vi "DMM6500_Soft_v0.vi"() -> ()   [LabVIEW 2023]
uses:
  Ctrl_state.ctl
  <vilib>/Instr/_visa.llb/VISA Find Search Mode.ctl
  <vilib>/Instr/_visa.llb/VISA Open Access Mode.ctl
  <vilib>/Utility/sysdir.llb/System Directory Type.ctl
  <instrlib>/Keithley DMM6500 DAQ6500 Series/Public/Data/Read (Multiple Points).vi
  <instrlib>/Keithley DMM6500 DAQ6500 Series/Keithley DMM6500 DAQ6500 Series.lvlib
panel:
  in  "Manual Range (1)":dbl=1.0 format="%#_13g"
  in  "Auto Range":bool=TRUE
  in  "Label":string="Sensor label"
  in  "NPLC":dbl(ring)=10.0 items=["0.01"=0.01, "0.1"=0.1, "1"=1.0, "5"=5.0, "10"=10.0, "25"=25.0, "50"=50.0]
  in  "Function (0: Voltage DC)":i32(ring)=4 items=["Voltage DC", "Voltage AC", "Current DC", "Current AC", "Resistance", "4-wire Resistance", "Diode", "Capacitance", "Temperature", "Continuity", "Frequency", "Period", "Voltage Ratio", "Digitize Voltage", "Digitize Current"]
  in  "Sensors":T1(array[cluster])
  in  "Meas":bool
  in  "Stop":bool
  out "Status":string
  out "Err/MSG":string
  in  "Tab Control":enum32{"Time Domain"}(tab)
  out "Data":cluster{dbl[], dbl[]}[](graph)
  # "Martin Hruska, 2026"
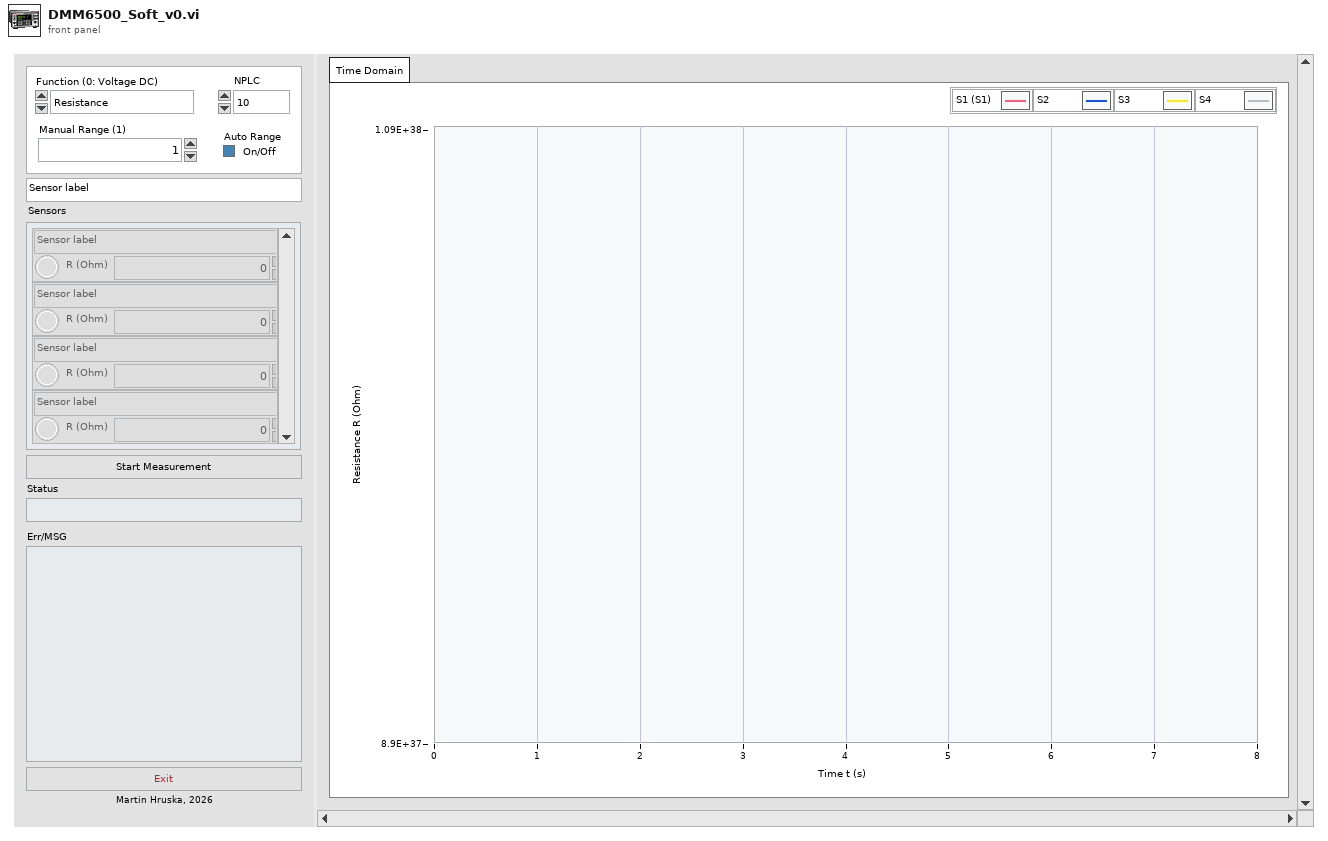
[diagram p1: front panel]
types:
  T1 = cluster{"S Label":string, "S On/Off":bool, "R (Ohm)":dbl}[]
  T2 = typedef "Ctrl_state.ctl" = enum16{"Initialize", "Wait", "Close", "Continuous"}
  T3 = enum8{"Enabled", "Disabled", "Disabled and Grayed Out"}
  T4 = enum16{"open", "replace", "create", "open or create", "replace or create", "replace or create with confirmation"}
  T5 = typedef "VISA Find Search Mode.ctl" = u32
  T6 = typedef "VISA Open Access Mode.ctl" = u32
  T7 = typedef "System Directory Type.ctl" = i32
  T8 = cluster{"S Label":string, "S On/Off":bool, "R (Ohm)":dbl}
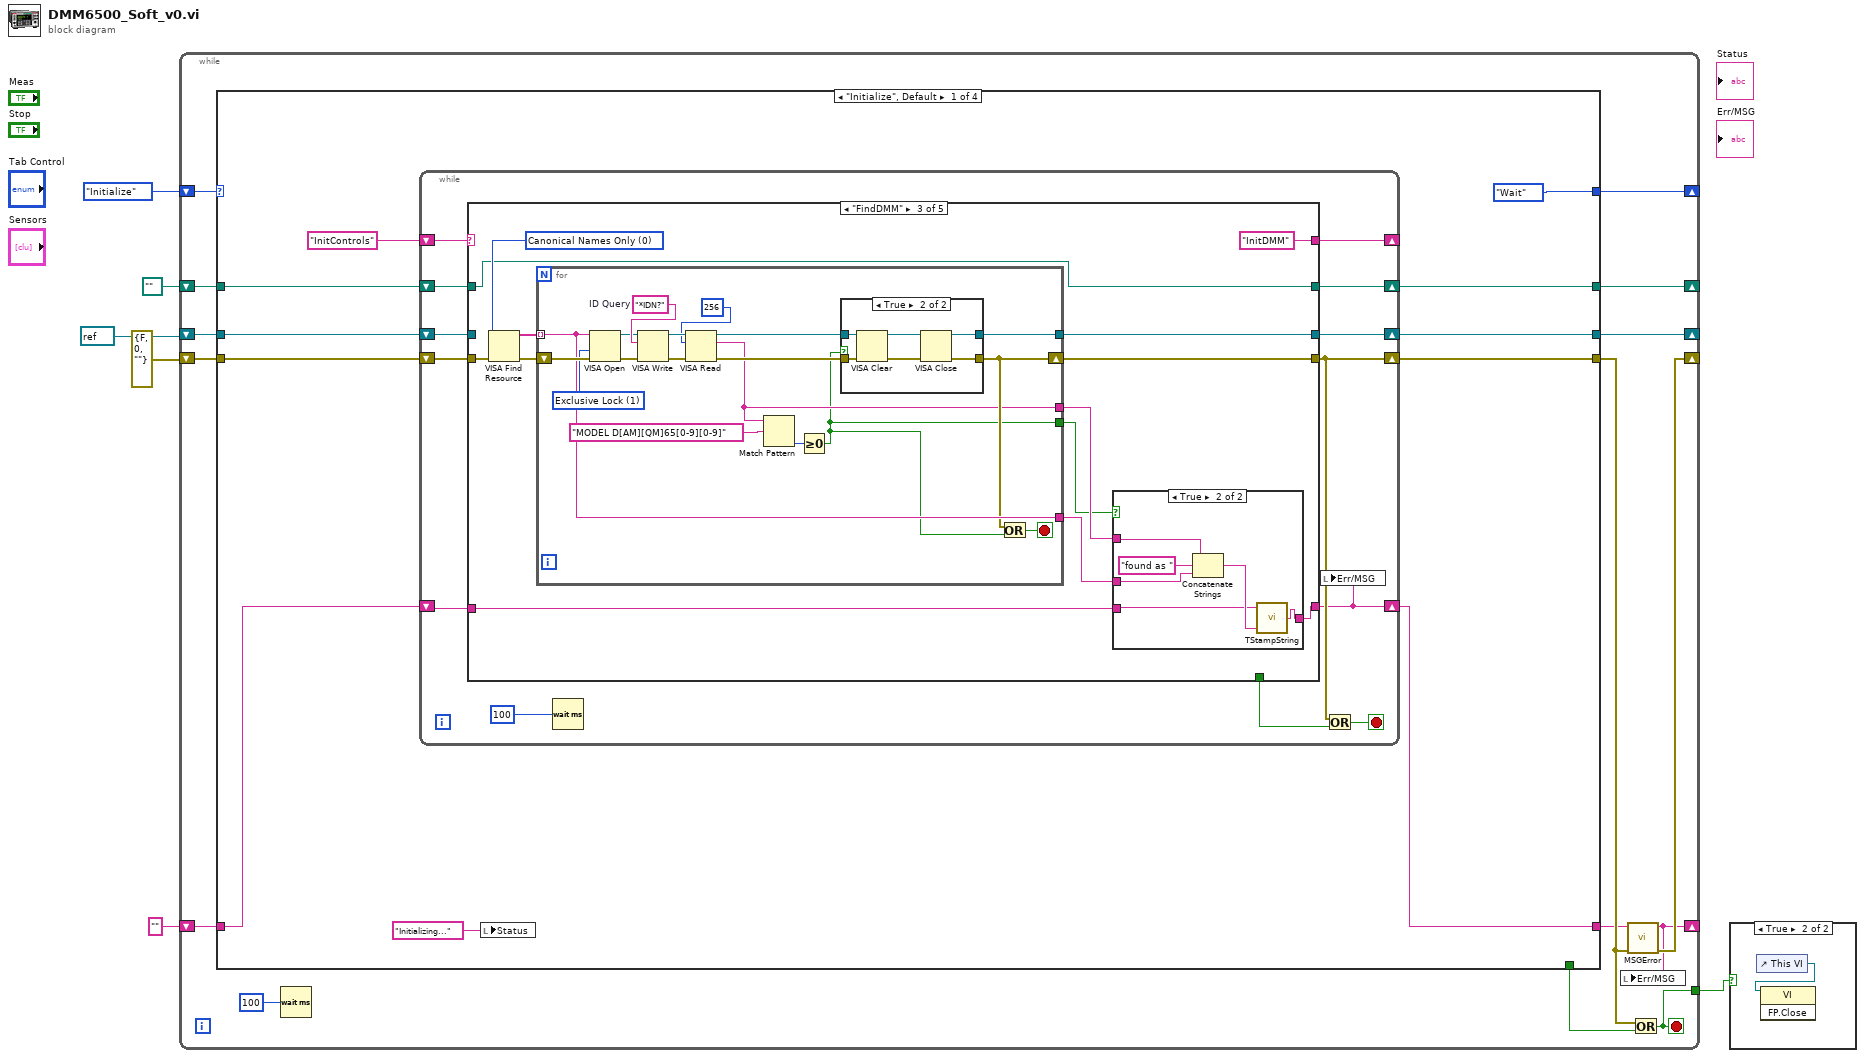
[diagram p0: block diagram]
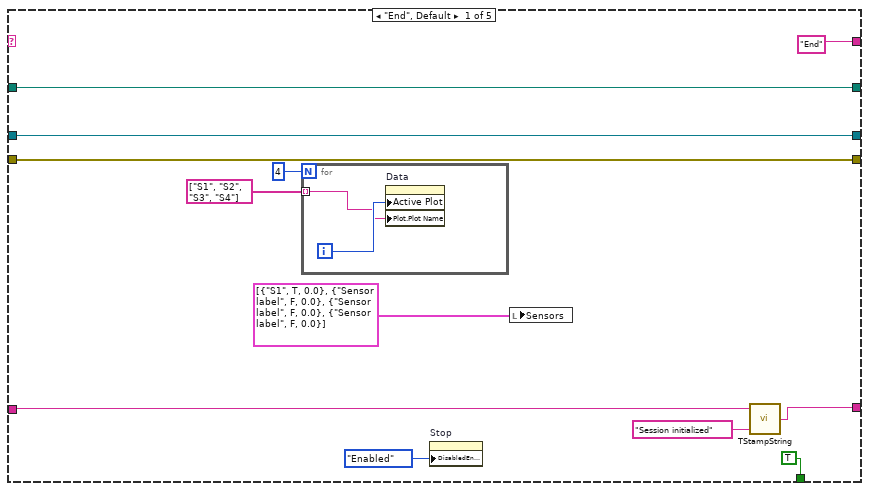
[diagram p3: hidden frame]
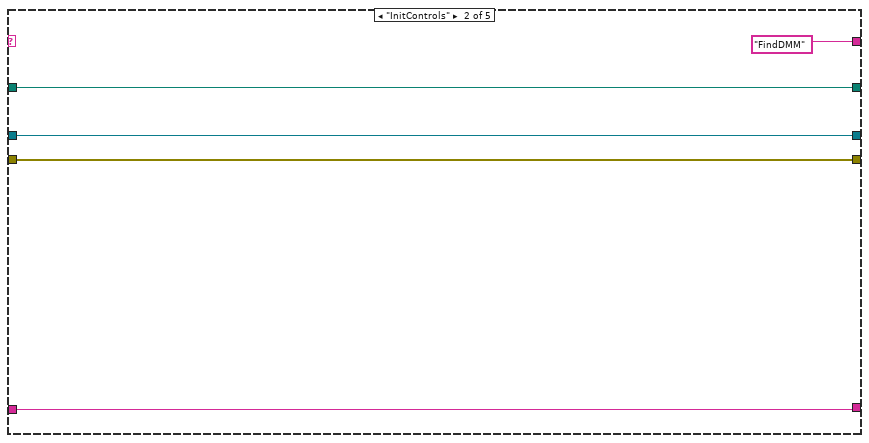
[diagram p4: hidden frame]
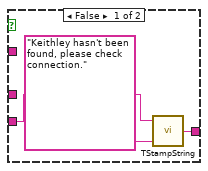
[diagram p5: hidden frame]
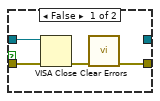
[diagram p6: hidden frame]
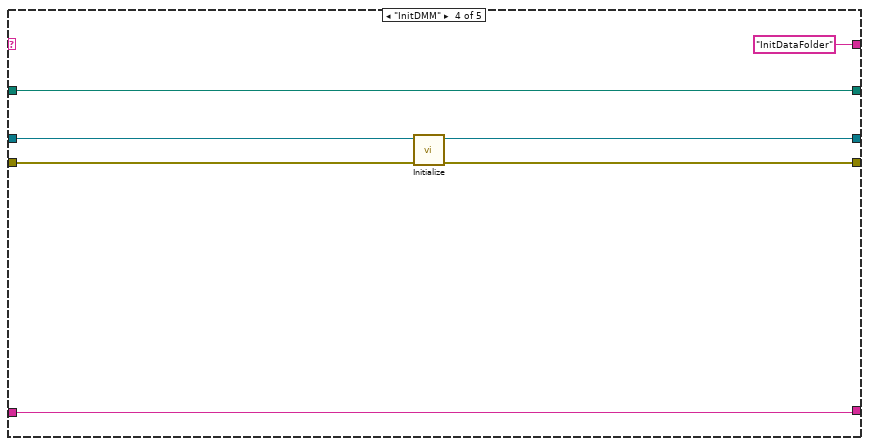
[diagram p7: hidden frame]
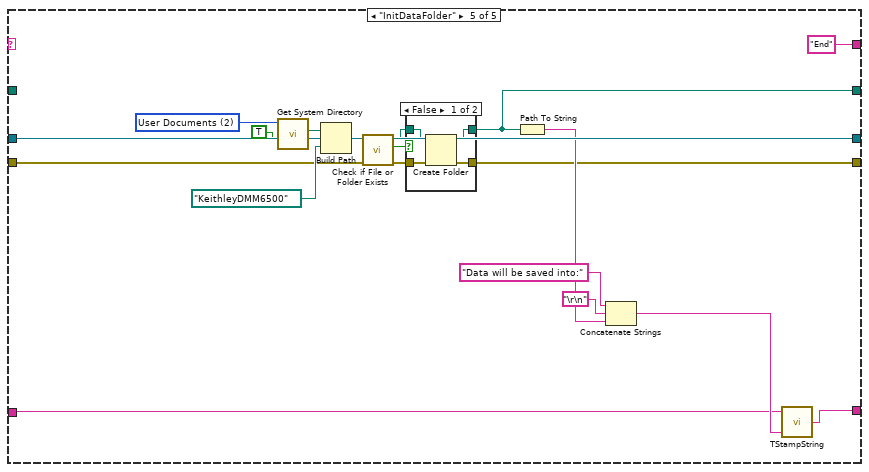
[diagram p8: hidden frame]
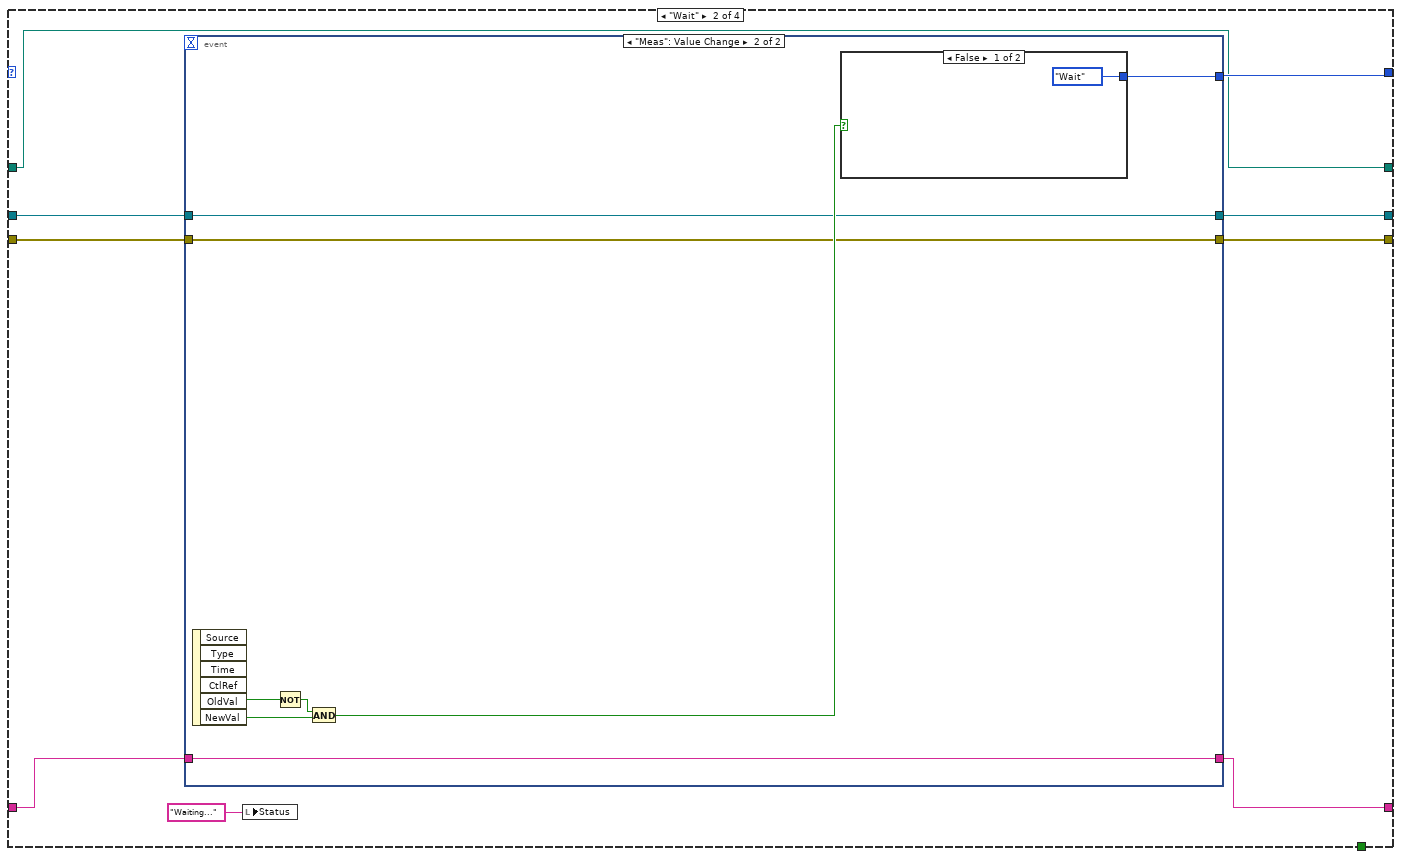
[diagram p10: hidden frame]
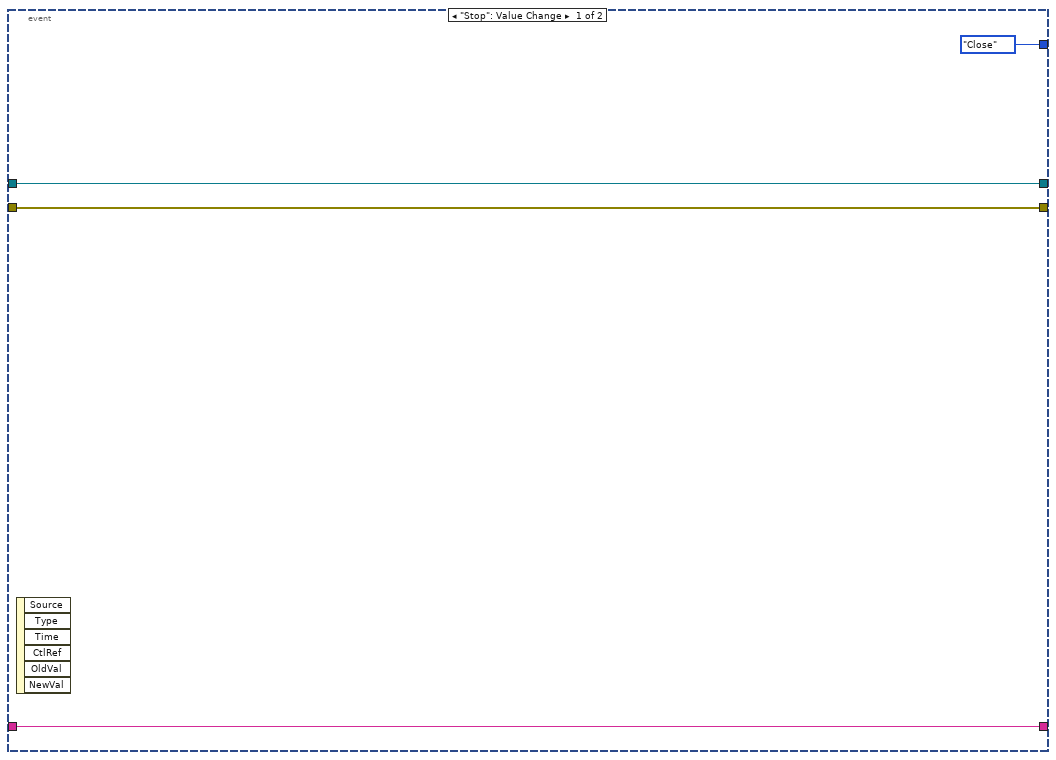
[diagram p11: hidden frame]
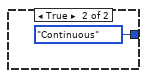
[diagram p12: hidden frame]
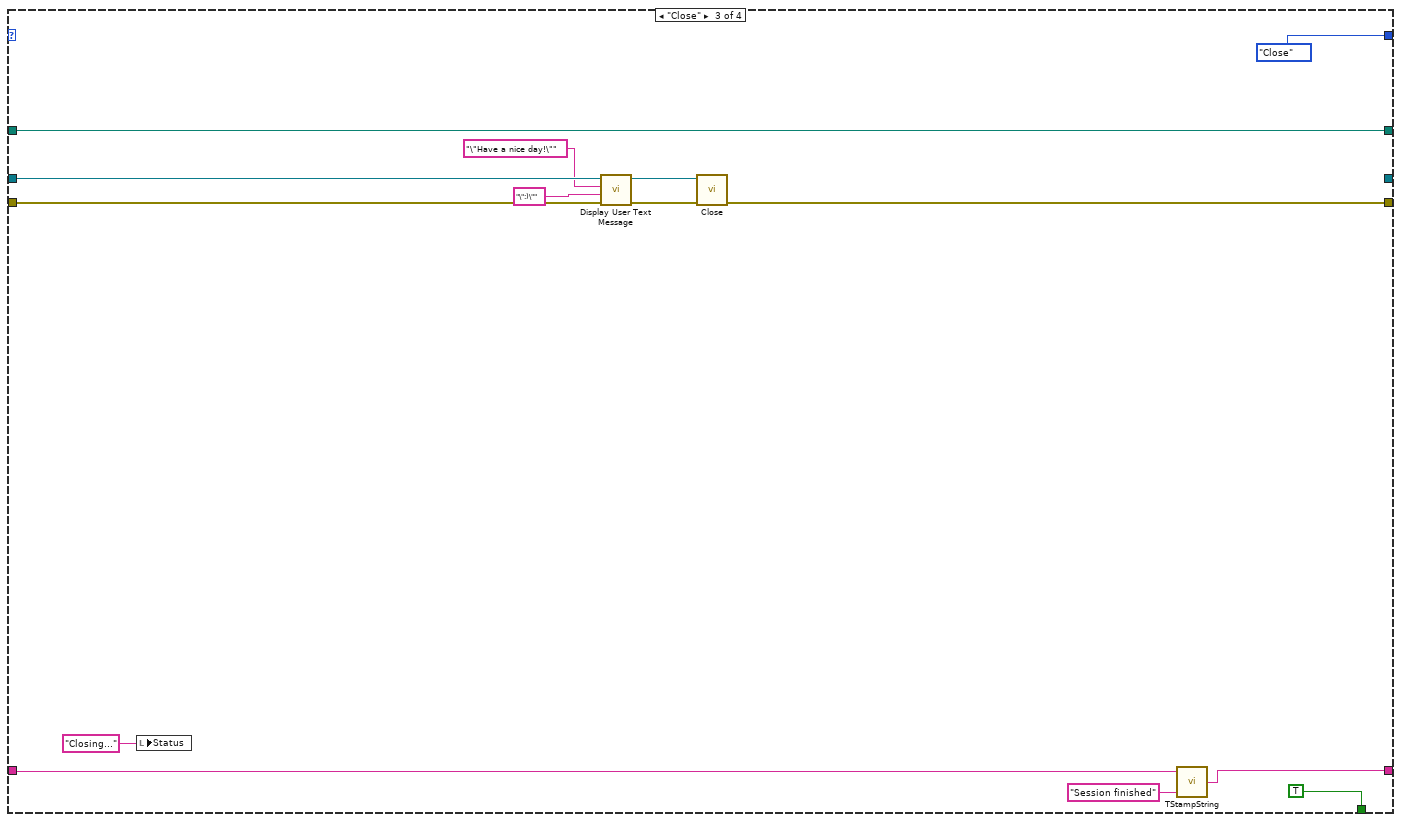
[diagram p13: hidden frame]
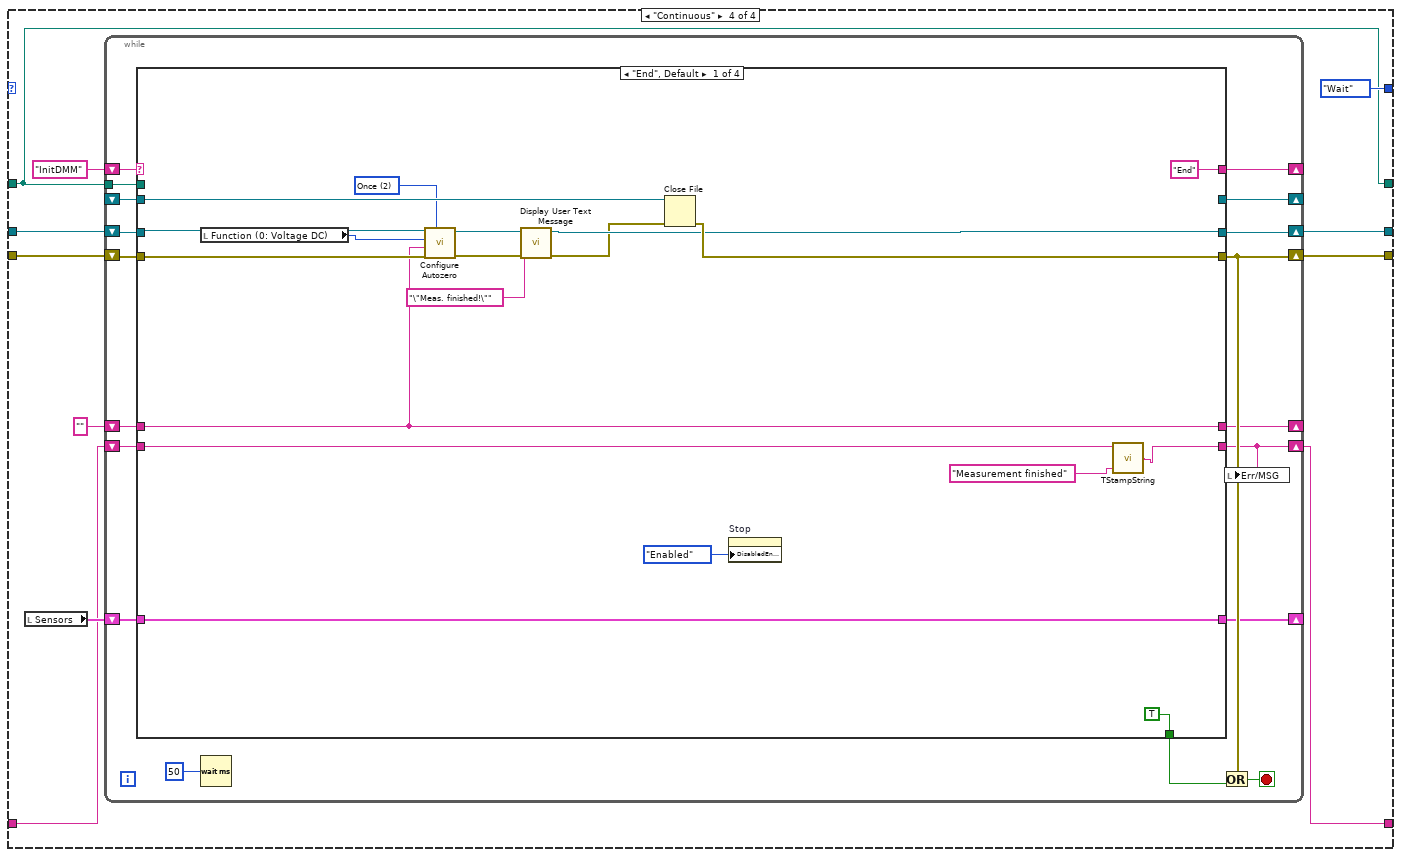
[diagram p14: hidden frame]
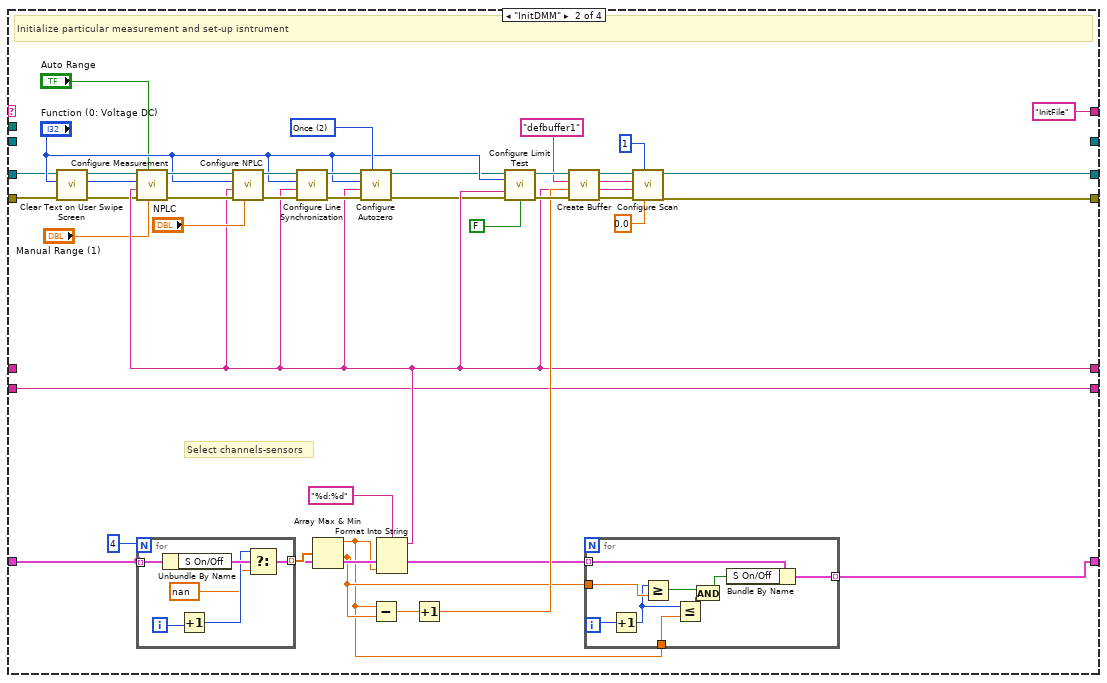
[diagram p15: hidden frame]
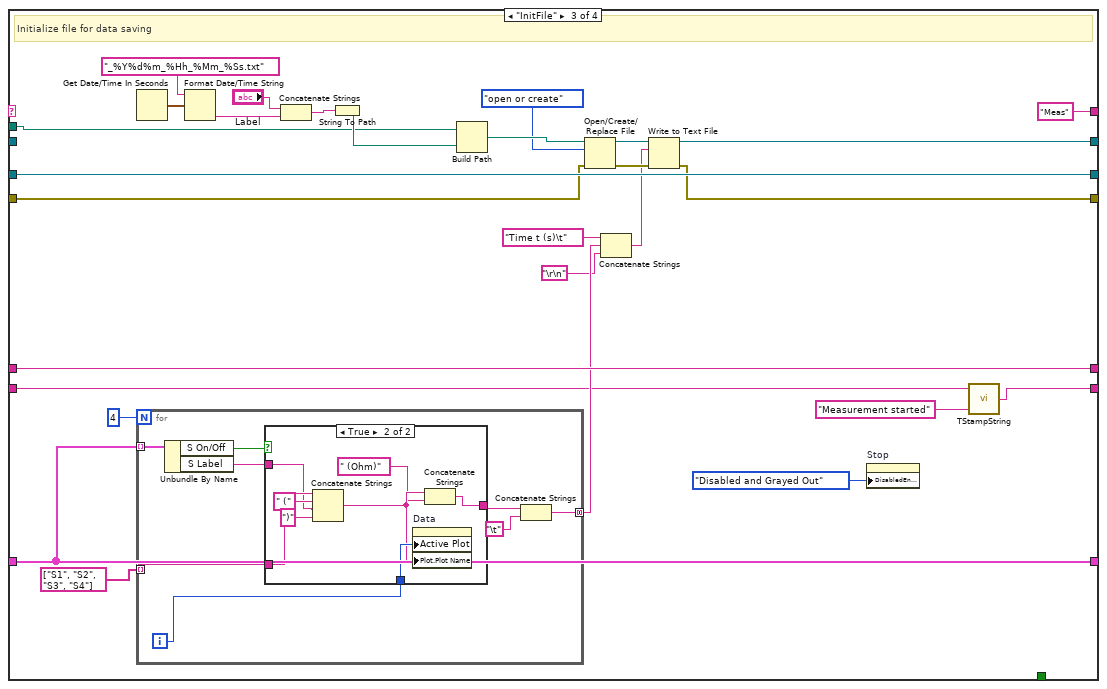
[diagram p16: hidden frame]
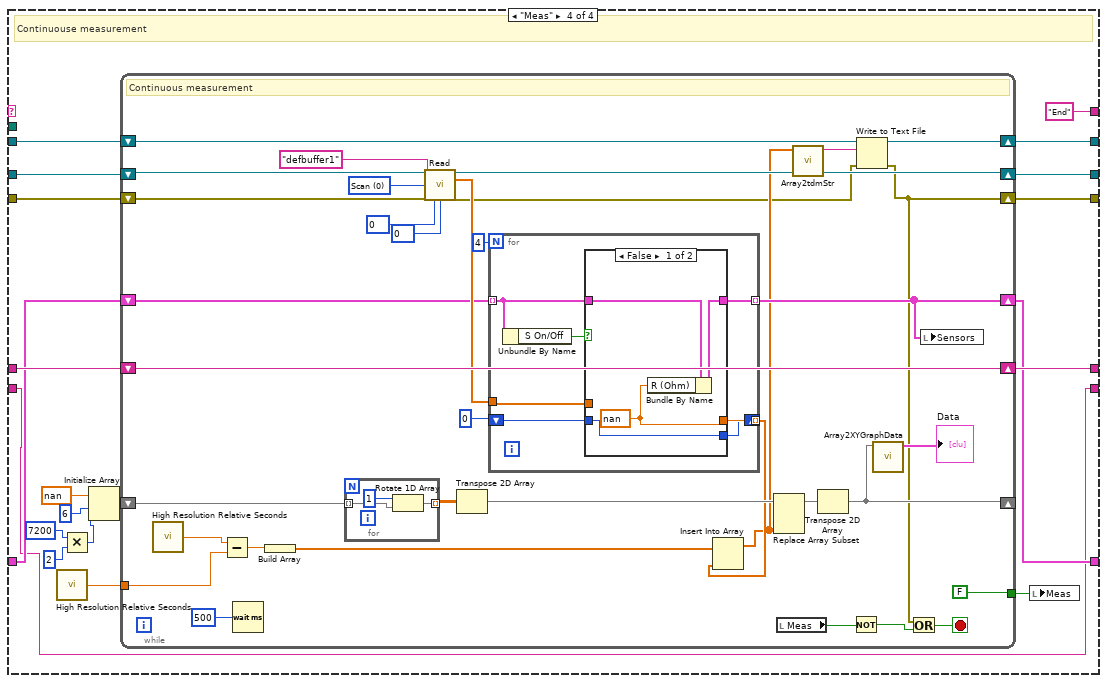
[diagram p18: hidden frame]
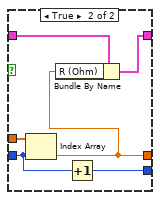
[diagram p19: hidden frame]
diagram:
  n1 = while {
    shift-right: [w20] -> _
    shift-left: Ctrl_state."Initialize" -> [w21]
    shift-right: [w16] -> _
    shift-left: errorcluster {"status"=FALSE, "code"=0, "source"=""} ("error constant") -> [w19]
    shift-right: [w11] -> _
    shift-left: "" ("OutputString") -> [w13]
    shift-right: [w12] -> _
    shift-left: refnum<visa-resource-name> refnum ("VISA resource name") -> [w18]
    shift-right: [w9] -> _
    shift-left: path "" ("dup path") -> [w8]
    tunnel: [w7] -> w1
    stop <- w7 stop-if-true
    n2 = case shown="\"Initialize\", Default" w21 {
      tunnel: [Ctrl_state."Wait" w154 Ctrl_state."Close" Ctrl_state."Wait"] -> w20
      tunnel: w19 -> [w30 w150 w175 w190]
      tunnel: w18 -> [w29 w148 w174 w189]
      tunnel: [_ _ TRUE _] -> w17
      tunnel: [w28 w151 w180 w191] -> w15
      tunnel: [w26 w152 w169 w183] -> w14
      tunnel: w13 -> [w27 w153 w170 w184]
      tunnel: [w25 w149 _ w188] -> w12
      tunnel: [w23 w146 w178 w185] -> w9
      tunnel: w8 -> [w22 w146 w178 w185]
      frame "Initialize", Default {
        n3 = while {
          shift-right: [w44] -> _
          shift-left: "InitControls" -> [w45]
          shift-right: [w39] -> w28
          shift-left: w30 -> [w40]
          shift-right: [w38] -> w25
          shift-left: w29 -> [w37]
          shift-right: [w35] -> w26
          shift-left: w27 -> [w36]
          shift-right: [w34] -> w23
          shift-left: w22 -> [w33]
          stop <- w42 stop-if-true
          n4 = case shown="\"FindDMM\"" w45 {
            tunnel: ["End" "FindDMM" "InitDMM" "InitDataFolder" "End"] -> w44
            tunnel: [TRUE _ _ _ _] -> w41
            tunnel: w40 -> [w54 w62 w73 w117 w126]
            tunnel: [w54 w62 w72 w116 w125] -> w39
            tunnel: [w55 w63 w71 w115 w138] -> w38
            tunnel: w37 -> [w55 w63 _ w118 w138]
            tunnel: w36 -> [w48 w61 w67 w120 w122]
            tunnel: [w46 w61 w66 w120 w121] -> w35
            tunnel: [w52 w60 w65 w114 w124] -> w34
            tunnel: w33 -> [w52 w60 w65 w114 _]
            frame "End", Default {
              n5 = for {
                N: 4 -> [_]
                tunnel: string[] ["S1", "S2", "S3", "S4"] -> [w58] mode=indexing
                i -> [w59]
                n6 = property on="Data" class="XYGraph (strict)"("Active Plot"=w59, "Plot.Plot Name"=w58) -> ()  [unwired: 2 in, 2 out]
              }
              n7 = property on="Stop" class="Bool"("DisabledEnum"=T3."Enabled" ("Disabled")) -> ()  [unwired: 2 in, 2 out]
              n8 = local write "Sensors"(T1 [{"S Label"="S1", "S On/Off"=TRUE, "R (Ohm)"=0.0}, {"S Label"="Sensor label", "S On/Off"=FALSE, "R (Ohm)"=0.0}, {"S Label"="Sensor label", "S On/Off"=FALSE, "R (Ohm)"=0.0}, {"S Label"="Sensor label", "S On/Off"=FALSE, "R (Ohm)"=0.0}] ("Sensors")) -> ()
              n9 = call "TStampString.vi"("Incoming string"="Session initialized", "Previous string"=w48) -> ("String with time stamp"=w46:string)  [unwired: 1 in]
            }
            frame "InitControls" {
            }
            frame "FindDMM" {
              w74 = T5 0 items=["Canonical Names Only"=0, "Aliases Only"=2, "Include Matching Aliases"=3, "Include All Aliases"=4] ("Search Mode")
              n10 = VISA Find Resource(8:w73, 10:w74) -> (0:w76:errorcluster, 3:w75:string[])  [unwired: 1 in, 1 out]
              n11 = for {
                tunnel: w75 -> [w95] mode=indexing
                tunnel: [w89] -> w69
                tunnel: [w95] -> w68
                shift-right: [w91] -> w72
                shift-left: w76 -> [w97]
                tunnel: [w96] -> w71
                tunnel: [w90] -> w70
                stop <- w92 stop-if-true
                w87 = T6 1 items=["VISA Defaults"=0, "Exclusive Lock"=1, "Load Configured Settings"=4] ("Access Mode")
                w104 = "*IDN?"  # ID Query
                n12 = VISA Open(access mode=w87, error in (no error)=w97, VISA resource name=w95) -> (VISA resource name=w101:refnum<visa-resource-name>, error out=w100:errorcluster)  [unwired: 2 in]
                n13 = VISA Write(VISA resource name=w101, write buffer=w104, error in (no error)=w100) -> (VISA resource name out=w103:refnum<visa-resource-name>, error out=w99:errorcluster)  [unwired: 1 out]
                n14 = VISA Read(VISA resource name=w103, byte count=u32 256, error in (no error)=w99) -> (VISA resource name out=w98:refnum<visa-resource-name>, read buffer=w90:string, error out=w93:errorcluster)  [unwired: 1 out]
                n15 = Match Pattern(string=w90, regular expression="MODEL D[AM][QM]65[0-9][0-9]") -> (offset past match=w94:i32)  [unwired: 1 in, 3 out]
                n16 = Greater Or Equal To 0?(x=w94) -> (x >= 0?=w89:bool)
                n17 = case shown="True" w89 {
                  tunnel: w98 -> [w108 w113]
                  tunnel: w93 -> [w107 w112]
                  tunnel: [w105 w109] -> w91
                  tunnel: [_ w111] -> w96
                  frame False {
                    n18 = VISA Close(VISA resource name=w108, error in (no error)=w107) -> (error out=w106:errorcluster)
                    n19 = call <vilib>:"Clear Errors.vi"("error in (no error)"=w106) -> ("error out"=w105:errorcluster)  [unwired: 5 in, 1 out]
                  }
                  frame True {
                    n20 = VISA Clear(VISA resource name=w113, error in (no error)=w112) -> (VISA resource name out=w111:refnum<visa-resource-name>, error out=w110:errorcluster)
                    n21 = VISA Close(VISA resource name=w111, error in (no error)=w110) -> (error out=w109:errorcluster)
                  }
                }
                n22 = Or(x=w91, y=w89) -> (x .or. y?=w92:bool)
              }
              n23 = case shown="True" w69 {
                tunnel: w67 -> [w80 w82]
                tunnel: w68 -> [_ w85]
                tunnel: [w78 w81] -> w66
                tunnel: w70 -> [_ w84]
                frame False {
                  n24 = call "TStampString.vi"("Incoming string"="Keithley hasn't been found, please check connection.", "Previous string"=w80) -> ("String with time stamp"=w78:string)  [unwired: 1 in]
                }
                frame True {
                  n25 = Concatenate Strings(w84, "found as " ("string"), w85) -> (w83:string)
                  n26 = call "TStampString.vi"("Incoming string"=w83, "Previous string"=w82) -> ("String with time stamp"=w81:string)  [unwired: 1 in]
                }
              }
            }
            frame "InitDMM" {
              n27 = call <instrlib>:"Initialize.vi"("error in (no error)"=w117, "VISA resource name"=w118) -> ("error out"=w116:errorcluster, "VISA resource name out"=w115:refnum<visa-resource-name>)  [unwired: 8 in]
            }
            frame "InitDataFolder" {
              w129 = T7 2 items=["User Home"=0, "User Desktop"=1, "User Documents"=2, "User Application Data"=3, "User Preferences"=4, "User Temporary"=5, "Public Documents"=6, "Public Application Data"=7, "Public Preferences"=8, "Public Cache"=13, "System Core Libraries"=9, "System Installed Libraries"=10, "Application Files"=11, "Boot Volume Root"=12] ("system directory type")
              n28 = call <vilib>:"Get System Directory.vi"("create directory if not found? (F)"=TRUE, "system directory type"=w129) -> ("system directory"=w127:path)  [unwired: 9 in]
              n29 = Build Path(base path=w127, name or relative path=path "KeithleyDMM6500") -> (appended path=w137:path)
              n30 = call <vilib>:"Check if File or Folder Exists.vi"("error in (no error)"=w126, "path"=w137) -> ("error out"=w134:errorcluster, "file or folder exists?"=w136:bool, "dup path"=w135:path)  [unwired: 7 in]
              n31 = case shown="False" w136 {
                tunnel: w135 -> [w143 w145]
                tunnel: w134 -> [w142 w144]
                tunnel: [w141 w145] -> w124
                tunnel: [w140 w144] -> w125
                frame False {
                  n32 = Create Folder(path (use dialog)=w143, error in=w142) -> (created path=w141:path, error out=w140:errorcluster)  [unwired: 1 in, 1 out]
                }
                frame True {
                }
              }
              n33 = Path To String(path=w124) -> (string=w131:string)
              n34 = Concatenate Strings("Data will be saved into:" ("string"), "\r\n", w131) -> (w123:string)
              n35 = call "TStampString.vi"("Incoming string"=w123, "Previous string"=w122) -> ("String with time stamp"=w121:string)  [unwired: 1 in]
            }
          }
          n36 = Wait (ms)(milliseconds to wait=u32 100) -> ()  [unwired: 1 out]
          n37 = local write "Err/MSG"(w35) -> ()
          n38 = Or(x=w39, y=w41) -> (x .or. y?=w42:bool)
        }
        n39 = local write "Status"("Initializing..." ("Status")) -> ()
      }
      frame "Wait" {
        n40 = event shown="[1] \"Meas\": Value Change" {
          selector: _ -> [_ _]
          dyn-events: _ -> [_ _]
          timeout: _ -> [_ _]
          tunnel: [Ctrl_state."Close" w166] -> w154
          tunnel: w153 -> [w157 w159]
          tunnel: [w157 w159] -> w152
          tunnel: [w156 w160] -> w151
          tunnel: w150 -> [w156 w160]
          tunnel: [w155 w161] -> w149
          tunnel: w148 -> [w155 w161]
          event "Stop": Value Change {
            n41 = event-data() -> ()  [unwired: 1 in, 6 out]
          }
          event "Meas": Value Change {
            n42 = event-data() -> ("OldVal"=w165:bool, "NewVal"=w163:bool)  [unwired: 1 in, 4 out]
            n43 = Not(x=w165) -> (.not. x?=w164:bool)
            n44 = And(x=w164, y=w163) -> (x .and. y?=w162:bool)
            n45 = case shown="False" w162 {
              tunnel: [Ctrl_state."Wait" Ctrl_state."Continuous"] -> w166
              frame False {
              }
              frame True {
              }
            }
          }
        }
        n46 = local write "Status"("Waiting..." ("Status")) -> ()
      }
      frame "Close" {
        n47 = local write "Status"("Closing..." ("Status")) -> ()
        n48 = call <instrlib>:"Display User Text Message.vi"("error in (no error)"=w175, "Lower Message (\"Message\")"="\":)\"" ("Lower Message (\"Message\")"), "Upper Message (\"Default\")"="\"Have a nice day!\"" ("Upper Message (\"Default\")"), "VISA resource name"=w174) -> ("error out"=w176:errorcluster, "VISA resource name out"=w177:refnum<visa-resource-name>)  [unwired: 6 in]
        n49 = call <instrlib>:"Close.vi"("error in (no error)"=w176, "VISA resource name"=w177) -> ("error out"=w180:errorcluster)  [unwired: 9 in]
        n50 = call "TStampString.vi"("Incoming string"="Session finished", "Previous string"=w170) -> ("String with time stamp"=w169:string)  [unwired: 1 in]
      }
      frame "Continuous" {
        n51 = local read "Sensors"() -> (w186:T1)
        n52 = while {
          shift-right: [w210] -> _
          shift-left: "InitDMM" -> [w211]
          shift-right: [w203] -> w191
          shift-left: w190 -> [w209]
          shift-right: [w208] -> w188
          shift-left: w189 -> [w207]
          shift-right: [w202] -> _
          shift-left: "" -> [w201]
          shift-right: [w199] -> _
          shift-left: w186 -> [w200]
          tunnel: w185 -> [w198]
          shift-right: [w197] -> _
          shift-left: _ -> [w196]
          shift-right: [w194] -> w183
          shift-left: w184 -> [w195]
          stop <- w204 stop-if-true
          n53 = case shown="\"End\", Default" w211 {
            tunnel: ["End" "InitFile" "Meas" "End"] -> w210
            tunnel: [TRUE _ _ _] -> w205
            tunnel: [w226 w248 w299 w344] -> w203
            tunnel: w209 -> [w224 w234 w300 w347]
            tunnel: [w218 w249 w312 w343] -> w208
            tunnel: w207 -> [w225 w237 w312 w346]
            tunnel: [w222 w240 w310 w348] -> w202
            tunnel: w201 -> [w222 _ w310 w349]
            tunnel: w200 -> [w228 w245 w295 w334]
            tunnel: [w228 w244 w295 w333] -> w199
            tunnel: w198 -> [_ _ w302 _]
            tunnel: [_ _ w301 w332] -> w197
            tunnel: w196 -> [w227 _ _ w331]
            tunnel: w195 -> [w213 w231 w287 w330]
            tunnel: [w212 w231 w286 w330] -> w194
            frame "End", Default {
              w223 = u32 2 items=["Enable", "Disable", "Once"] ("Auto Zero (0: Enable)")
              n54 = local read "Function (0: Voltage DC)"() -> (w221:i32)
              n55 = call <instrlib>:"Configure Autozero.vi"("Auto Zero (0: Enable)"=w223, "error in (no error)"=w224, "Channel List(\"\")"=w222, "Function (0: Voltage DC)"=w221, "VISA resource name"=w225) -> ("error out"=w219:errorcluster, "VISA resource name out"=w220:refnum<visa-resource-name>)  [unwired: 5 in]
              n56 = call <instrlib>:"Display User Text Message.vi"("error in (no error)"=w219, "Upper Message (\"Default\")"="\"Meas. finished!\"" ("Upper Message (\"Default\")"), "VISA resource name"=w220) -> ("error out"=w217:errorcluster, "VISA resource name out"=w218:refnum<visa-resource-name>)  [unwired: 7 in]
              n57 = Close File(refnum=w227, error in=w217) -> (error out=w226:errorcluster)  [unwired: 1 out]
              n58 = property on="Stop" class="Bool"("DisabledEnum"=T3."Enabled" ("Disabled")) -> ()  [unwired: 2 in, 2 out]
              n59 = call "TStampString.vi"("Incoming string"="Measurement finished", "Previous string"=w213) -> ("String with time stamp"=w212:string)  [unwired: 1 in]
            }
            frame "InitDMM" {
              w252 = "defbuffer1" ("Reading Buffer (\"defbuffer1\")")
              w260 = u32 2 items=["Enable", "Disable", "Once"] ("Auto Zero (0: Enable)")
              # "Select channels-sensors"
              # "Initialize particular measurement and set-up isntrument"
              n60 = call <instrlib>:"Clear Text on User Swipe Screen.vi"("error in (no error)"=w234, "VISA resource name"=w237) -> ("error out"=w235:errorcluster, "VISA resource name out"=w236:refnum<visa-resource-name>)  [unwired: 8 in]
              n61 = for {
                N: 4 -> [_]
                tunnel: w245 -> [w284] mode=indexing
                tunnel: [w280] -> w268 mode=indexing
                i -> [w283]
                n62 = Unbundle By Name(w284) -> ("S On/Off"=w281:bool)
                n63 = Increment(x=w283) -> (x+1=w282:i32)
                n64 = Select(t=w282, s=w281, f=nan) -> (s? t:f=w280:dbl)
              }
              n65 = Array Max & Min(array=w268) -> (max value=w242:dbl, min value=w243:dbl)  [unwired: 2 out]
              n66 = Subtract(x=w242, y=w243) -> (x-y=w247:dbl)
              n67 = Format Into String(format string="%d:%d", w243, w242) -> (resulting string=w240:string)  [unwired: 2 in, 1 out]
              n68 = call <instrlib>:"Configure Measurement.vi"("Manual Range (1)"="Manual Range (1)", "Auto Range (T: Enable)"="Auto Range", "error in (no error)"=w235, "Channel List(\"\")"=w240, "Function (0: Voltage DC)"="Function (0: Voltage DC)", "VISA resource name"=w236) -> ("error out"=w265:errorcluster, "VISA resource name out"=w266:refnum<visa-resource-name>)  [unwired: 4 in]
              n69 = call <instrlib>:"Configure NPLC.vi"("Power Line Cycle (1)"="NPLC", "error in (no error)"=w265, "Channel List(\"\")"=w240, "Function (0: Voltage DC)"="Function (0: Voltage DC)", "VISA resource name"=w266) -> ("error out"=w263:errorcluster, "VISA resource name out"=w264:refnum<visa-resource-name>)  [unwired: 5 in]
              n70 = call <instrlib>:"Configure Line Synchronization.vi"("error in (no error)"=w263, "Channel List(\"\")"=w240, "Function (0: Voltage DC)"="Function (0: Voltage DC)", "VISA resource name"=w264) -> ("error out"=w261:errorcluster, "VISA resource name out"=w262:refnum<visa-resource-name>)  [unwired: 6 in]
              n71 = call <instrlib>:"Configure Autozero.vi"("Auto Zero (0: Enable)"=w260, "error in (no error)"=w261, "Channel List(\"\")"=w240, "Function (0: Voltage DC)"="Function (0: Voltage DC)", "VISA resource name"=w262) -> ("error out"=w238:errorcluster, "VISA resource name out"=w239:refnum<visa-resource-name>)  [unwired: 5 in]
              n72 = Increment(x=w247) -> (x+1=w246:dbl)
              n73 = call <instrlib>:"Configure Limit Test.vi"("VISA resource name"=w239, "Function (0: Voltage DC)"="Function (0: Voltage DC)", "Channel List(\"\")"=w240, "error in (no error)"=w238, "Enable Limit (F: Disable)"=FALSE) -> ("VISA resource name out"=w257:refnum<visa-resource-name>, "error out"=w256:errorcluster)  [unwired: 9 in]
              n74 = call <instrlib>:"Create Buffer.vi"("error in (no error)"=w256, "Buffer Size (10)"=w246, "Buffer Name (\"\")"=w252, "VISA resource name"=w257) -> ("error out"=w253:errorcluster, "VISA resource name out"=w254:refnum<visa-resource-name>)  [unwired: 6 in]
              n75 = for {
                tunnel: w245 -> [w278] mode=indexing
                tunnel: [w277] -> w244 mode=indexing
                tunnel: w243 -> [w275]
                tunnel: w242 -> [w273]
                i -> [w276]
                n76 = Increment(x=w276) -> (x+1=w274:i32)
                n77 = Greater Or Equal?(x=w274, y=w275) -> (x >= y?=w272:bool)
                n78 = Less Or Equal?(x=w274, y=w273) -> (x <= y?=w271:bool)
                n79 = And(x=w272, y=w271) -> (x .and. y?=w270:bool)
                n80 = Bundle By Name(cluster=w278, "S On/Off"=w270) -> (w277:T8)
              }
              n81 = call <instrlib>:"Configure Scan.vi"("Delay Seconds (0 s)"=0.0, "Scan Count (1)"=u32 1, "error in (no error)"=w253, "Channel List(\"\")"=w240, "Reading Buffer (\"\")"=w252, "VISA resource name"=w254) -> ("error out"=w248:errorcluster, "VISA resource name out"=w249:refnum<visa-resource-name>)  [unwired: 4 in]
            }
            frame "InitFile" {
              # "Initialize file for data saving"
              n82 = Get Date/Time In Seconds() -> (seconds since 1Jan1904=w304:timestamp)
              n83 = for {
                N: 4 -> [_]
                tunnel: w295 -> [w320] mode=indexing
                tunnel: [w314] -> w293 mode=concatenating
                tunnel: string[] ["S1", "S2", "S3", "S4"] -> [w313] mode=indexing
                i -> [w317]
                n84 = Unbundle By Name(w320) -> ("S On/Off"=w319:bool, "S Label"=w318:string)
                n85 = case shown="True" w319 {
                  tunnel: w313 -> [w321 w329]
                  tunnel: w318 -> [_ w327]
                  tunnel: w317 -> [_ w325]
                  tunnel: [w321 w322] -> w315
                  frame False {
                  }
                  frame True {
                    n86 = Concatenate Strings(w329, " (" ("string"), w327, ")" ("string")) -> (w324:string)
                    n87 = property on="Data" class="XYGraph (strict)"("Active Plot"=w325, "Plot.Plot Name"=w324) -> ()  [unwired: 2 in, 2 out]
                    n88 = Concatenate Strings(w324, " (Ohm)" ("string")) -> (w322:string)
                  }
                }
                n89 = Concatenate Strings(w315, "\t") -> (w314:string)
              }
              n90 = Format Date/Time String(time format string (%c)="_%Y%d%m_%Hh_%Mm_%Ss.txt", seconds (now)=w304) -> (date/time string=w297:string)  [unwired: 1 in]
              n91 = Concatenate Strings("Label", w297) -> (w305:string)
              n92 = String To Path(string=w305) -> (path=w306:path)
              n93 = Build Path(base path=w302, name or relative path=w306) -> (appended path=w307:path)
              n94 = Open/Create/Replace File(file path (use dialog)=w307, error in=w300, operation (0:open)=T4."open or create") -> (refnum out=w308:refnum<file>, error out=w309:errorcluster)  [unwired: 3 in, 1 out]
              n95 = Concatenate Strings("Time t (s)\t" ("string"), w293, "\r\n") -> (w290:string)
              n96 = Write to Text File(file (use dialog)=w308, text=w290, error in=w309) -> (refnum out=w301:refnum<file>, error out=w299:errorcluster)  [unwired: 1 in, 1 out]
              n97 = property on="Stop" class="Bool"("DisabledEnum"=T3."Disabled and Grayed Out" ("Disabled")) -> ()  [unwired: 2 in, 2 out]
              n98 = call "TStampString.vi"("Incoming string"="Measurement started", "Previous string"=w287) -> ("String with time stamp"=w286:string)  [unwired: 1 in]
            }
            frame "Meas" {
              # "Continuouse measurement"
              n99 = call <vilib>:"High Resolution Relative Seconds.vi"() -> ("relative seconds"=w341:dbl)
              n100 = Multiply(x=7200 ("dimension size"), y=2 ("dimension size")) -> (x*y=w338:i32)
              n101 = Initialize Array(nan ("element"), 6 ("dimension size"), w338) -> (w335:dbl[][])
              n102 = while {
                shift-right: [w372] -> w348
                shift-left: w349 -> [w372]
                shift-right: [w351] -> w344
                shift-left: w347 -> [w383]
                shift-right: [w377] -> w343
                shift-left: w346 -> [w382]
                tunnel: [FALSE] -> w342
                tunnel: w341 -> [w368]
                shift-right: [w356] -> _
                shift-left: w335 -> [w367]
                shift-right: [w359] -> w333
                shift-left: w334 -> [w360]
                shift-right: [w355] -> w332
                shift-left: w331 -> [w354]
                stop <- w384 stop-if-true
                w378 = 0 items=["", "Date", "Extra", "Formatted", "Fractional", "Reading", "Relative", "Seconds", "Status", "Time", "Tstamp", "Unit", "CHAN", "Extra Form", "Extra Unit"] ("Buffer Element2 ()")
                w379 = 0 items=["", "Date", "Extra", "Formatted", "Fractional", "Reading", "Relative", "Seconds", "Status", "Time", "Tstamp", "Unit", "CHAN", "Extra Format", "Extra Unit"] ("Buffer Element1 ()")
                w380 = 0 items=["Scan", "Trigger"] ("Capture Mode(0: Scan)")
                # "Continuous measurement"
                n103 = call <vilib>:"High Resolution Relative Seconds.vi"() -> ("relative seconds"=w369:dbl)
                n104 = Subtract(x=w369, y=w368) -> (x-y=w363:dbl)
                n105 = Wait (ms)(milliseconds to wait=u32 500) -> ()  [unwired: 1 out]
                n106 = Build Array(w363) -> (w362:dbl[])
                n107 = for {
                  tunnel: [w386] -> w366 mode=indexing
                  tunnel: w367 -> [w385] mode=indexing
                  n108 = Rotate 1D Array(1:w385, 2:1 ("n")) -> (0:w386:dbl[])
                }
                n109 = call-poly <instrlib>:"Read.vi"("VISA resource name"=w382, "Buffer Name (\"\")"="defbuffer1" ("Buffer Name (\"\")"), "Capture Mode(0: Scan)"=w380, "error in (no error)"=w383, "Buffer Element1 ()"=w379, "Buffer Element2 ()"=w378) -> ("VISA resource name out"=w377:refnum<visa-resource-name>, "Measurements"=w371:dbl[], "error out"=w350:errorcluster)  [unwired: 7 in]
                n110 = Transpose 2D Array(2D array=w366) -> (transposed array=w365:dbl[][])
                n111 = for {
                  N: 4 -> [_]
                  tunnel: w371 -> [w394]
                  tunnel: [w393] -> w361 mode=indexing
                  tunnel: w360 -> [w391] mode=indexing
                  tunnel: [w392] -> w359 mode=indexing
                  shift-right: [w388] -> _
                  shift-left: 0 -> [w389]
                  n112 = Unbundle By Name(w391) -> ("S On/Off"=w390:bool)
                  n113 = case shown="False" w390 {
                    tunnel: w394 -> [_ w404]
                    tunnel: [w398 w403] -> w393
                    tunnel: w391 -> [w397 w401]
                    tunnel: [w396 w402] -> w392
                    tunnel: w389 -> [w395 w400]
                    tunnel: [w395 w399] -> w388
                    frame False {
                      w398 = nan
                      n114 = Bundle By Name(cluster=w397, "R (Ohm)"=w398) -> (w396:T8)
                    }
                    frame True {
                      n115 = Index Array(array=w404, index=w400) -> (element=w403:dbl)
                      n116 = Bundle By Name(cluster=w401, "R (Ohm)"=w403) -> (w402:T8)
                      n117 = Increment(x=w400) -> (x+1=w399:i32)
                    }
                  }
                }
                n118 = Insert Into Array(array=w362, new element=w361) -> (w352:dbl[])  [unwired: 1 in]
                n119 = Replace Array Subset(array=w365, new element=w352) -> (w364:dbl[][])  [unwired: 2 in]
                n120 = local read "Meas"() -> (w376:bool)
                n121 = call "Array2tdmStr.vi"("Array"=w352) -> ("String"=w353:string)  [unwired: 10 in]
                n122 = Transpose 2D Array(2D array=w364) -> (transposed array=w356:dbl[][])
                n123 = Not(x=w376) -> (.not. x?=w375:bool)
                n124 = Write to Text File(file (use dialog)=w354, text=w353, error in=w350) -> (refnum out=w355:refnum<file>, error out=w351:errorcluster)  [unwired: 1 in, 1 out]
                n125 = call "Array2XYGraphData.vi"("Array in"=w356) -> ("Array out"=→"Data":cluster{dbl[], dbl[]}[])  [unwired: 10 in]
                n126 = Or(x=w351, y=w375) -> (x .or. y?=w384:bool)
                n127 = local write "Sensors"(w359) -> ()
              }
              n128 = local write "Meas"(w342) -> ()
            }
          }
          n129 = Wait (ms)(milliseconds to wait=u32 50) -> ()  [unwired: 1 out]
          n130 = Or(x=w203, y=w205) -> (x .or. y?=w204:bool)
          n131 = local write "Err/MSG"(w194) -> ()
        }
      }
    }
    n132 = Wait (ms)(milliseconds to wait=u32 100) -> ()  [unwired: 1 out]
    n133 = call "MSGError.vi"("error in (no error)"=w15, "IncomingString"=w14) -> ("error out"=w16:errorcluster, "OutputString"=w11:string)  [unwired: 8 in]
    n134 = local write "Err/MSG"(w11) -> ()
    n135 = Or(x=w15, y=w17) -> (x .or. y?=w7:bool)
  }
  n136 = case shown="True" w1 {
    frame False {
    }
    frame True {
      n137 = control-ref of="This VI"() -> (w405:refnum<vi>)
      n138 = invoke class="VI" method="FP.Close"(reference=w405) -> ()  [unwired: 2 in, 3 out]
    }
  }
